vi "KT15 UP & DOWN.vi"() -> ()   [LabVIEW 2016]
uses:
  <vilib>/Instr/_visa.llb/VISA Configure Serial Port (Instr).vi
panel:
  in  "flow control 2":u16(ring) items=["None"=0, "XON/XOFF"=1, "RTS/CTS"=2, "DTR/DSR"=4]
  in  "stop bits 2":u16(ring)=10 items=["1.0"=10, "1.5"=15, "2.0"=20]
  in  "parity 2":u16(ring) items=["None", "Odd", "Even", "Mark", "Space"]
  in  "data bits 2":u16=8 min=5 max=8 step=1
  in  "KT-15 SKY":refnum<visa-resource-name>="COM17"
  in  "baud rate 2":u32=19200 min=2400 max=19200 step=2400
  out "KT-15 SKY Ambient Temperature":string
  out "KT-15 SKY  Temperature":string
  in  "Start or Stop Program":bool=TRUE
  out "KT-15 SEA Ambient Temperature":string
  out "KT-15 SEA Temperature":string
  in  "flow control":u16(ring) items=["None"=0, "XON/XOFF"=1, "RTS/CTS"=2, "DTR/DSR"=4]
  in  "stop bits":u16(ring)=10 items=["1.0"=10, "1.5"=15, "2.0"=20]
  in  "parity":u16(ring) items=["None", "Odd", "Even", "Mark", "Space"]
  in  "data bits":u16=8 min=5 max=8 step=1
  in  "KT-15 SEA":refnum<visa-resource-name>="COM16"
  in  "baud rate":u32=19200 min=2400 max=19200 step=2400
  # "COMM Port settings"
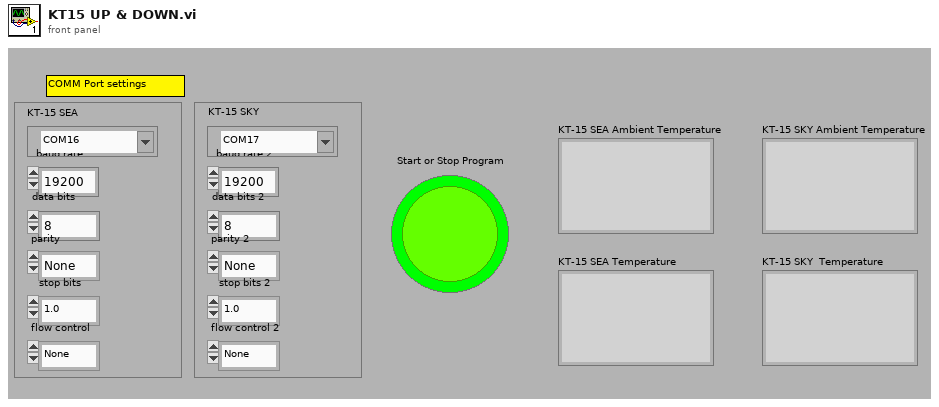
[diagram p1: front panel]
types:
  T1 = enum16{"open", "replace", "create", "open or create", "replace or create", "replace or create with confirmation"}
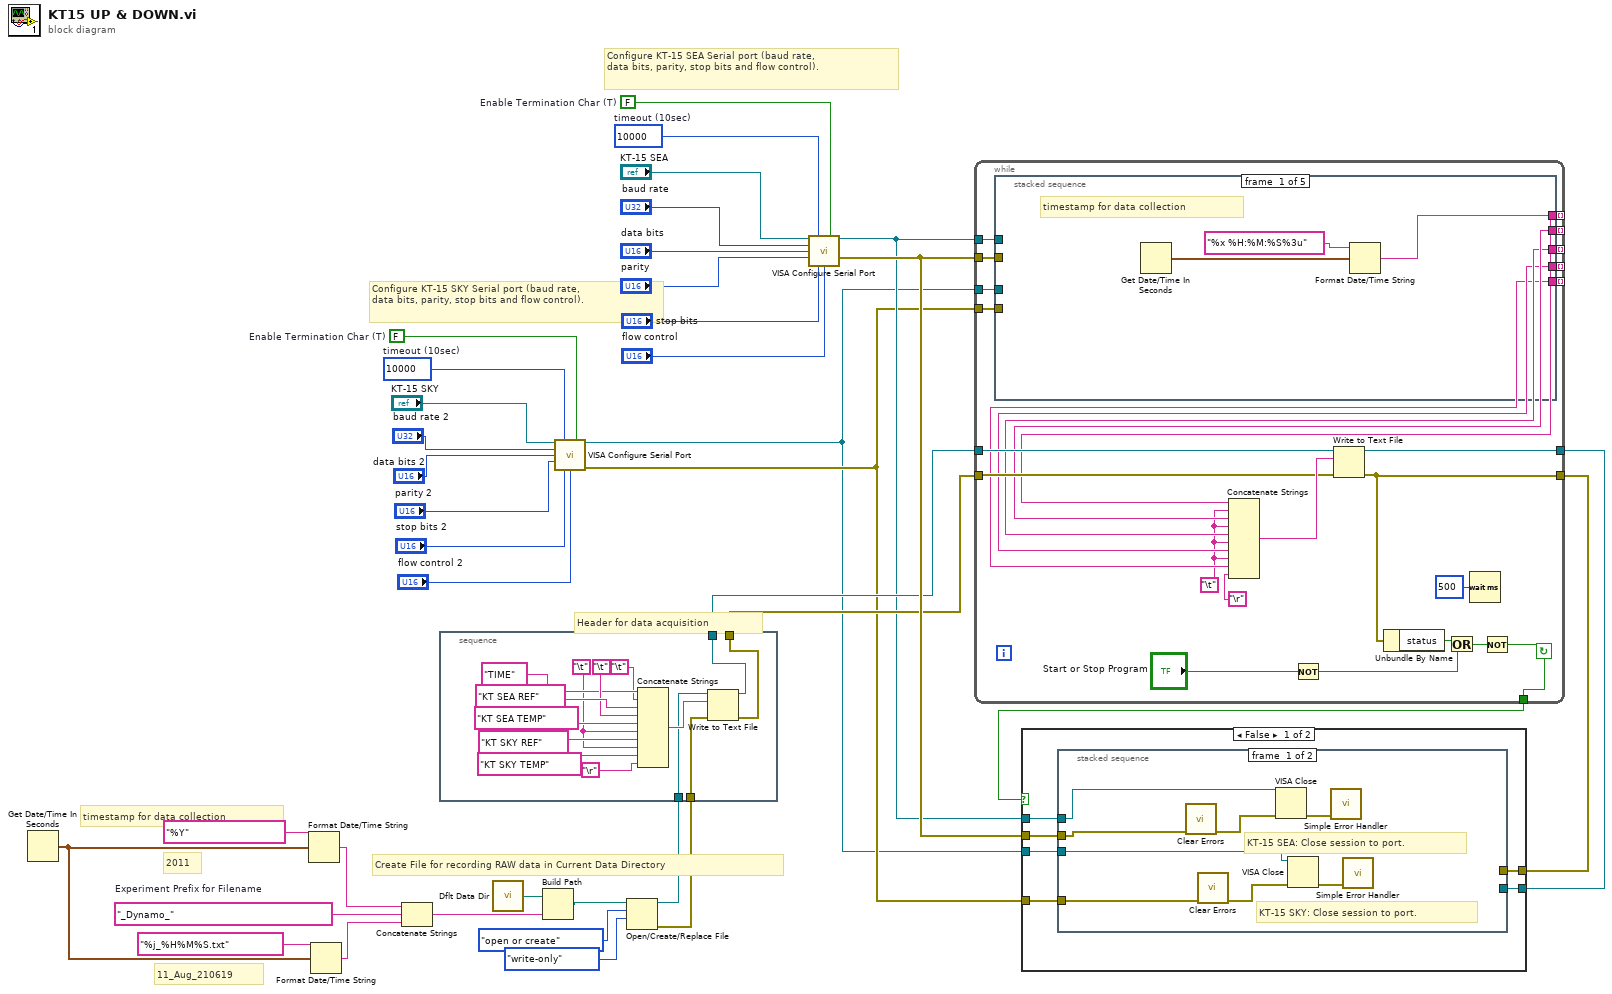
[diagram p0: block diagram]
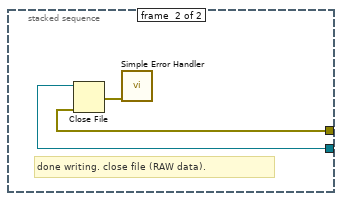
[diagram p2: hidden frame]
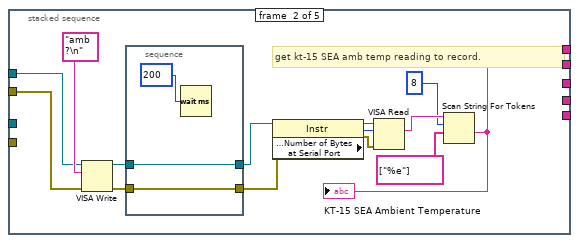
[diagram p4: hidden frame]
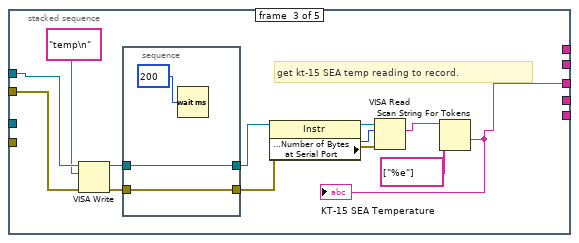
[diagram p5: hidden frame]
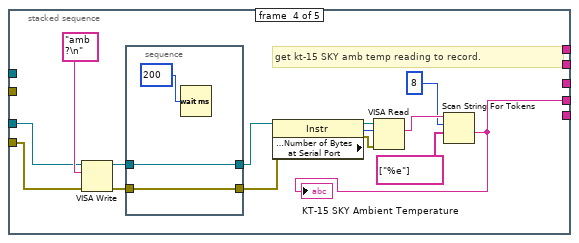
[diagram p6: hidden frame]
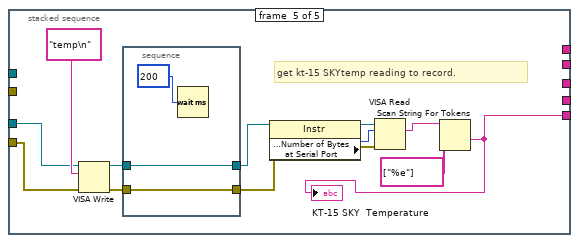
[diagram p7: hidden frame]
diagram:
  w19 = FALSE  # Enable Termination Char (T)
  w18 = u32 10000  # timeout (10sec)
  w8 = "_Dynamo_"  # Experiment Prefix for Filename
  w34 = FALSE  # Enable Termination Char (T)
  w35 = u32 10000  # timeout (10sec)
  # "2011"
  # "11_Aug_210619"
  # "timestamp for data collection"
  # "Configure KT-15 SKY Serial port (baud rate,\ndata bits, parity, stop bits and flow control)."
  # "Header for data acquisition"
  # "Create File for recording RAW data in Current Data Directory"
  # "Configure KT-15 SEA Serial port (baud rate,\ndata bits, parity, stop bits and flow control)."
  n1 = Get Date/Time In Seconds() -> (seconds since 1Jan1904=w5:timestamp)
  n2 = Format Date/Time String(time format string (%c)="%Y", seconds (now)=w5) -> (date/time string=w4:string)  [unwired: 1 out]
  n3 = Format Date/Time String(time format string (%c)="%j_%H%M%S.txt", seconds (now)=w5) -> (date/time string=w7:string)  [unwired: 1 out]
  n4 = Concatenate Strings(w4, w8, w7) -> (w1:string)
  n5 = call <vilib>:"Dflt Data Dir.vi"() -> ("App:Default Data Directory"=w3:path)
  n6 = Build Path(base path=w3, name or relative path=w1) -> (appended path=w2:path)
  n7 = call-poly "VISA Configure Serial Port"("VISA resource name"="KT-15 SKY", "timeout (10sec)"=w18, "Enable Termination\nChar (T)"=w19, "baud rate (9600)"="baud rate 2", "data bits (8)"="data bits 2", "parity (0:none)"="parity 2", "stop bits (10: 1 bit)"="stop bits 2", "flow control (0:none)"="flow control 2") -> ("VISA resource name out"=w10:refnum<visa-resource-name>, "error out"=w11:errorcluster)  [unwired: 1 in, 5 out]
  n8 = Open/Create/Replace File(file path (use dialog)=w2, operation (0:open)=T1."open or create", access (0:read/write)=enum16{"read/write", "read-only", "write-only"}."write-only") -> (refnum out=w28:refnum<file>, error out=w27:errorcluster)  [unwired: 3 in, 1 out]
  n9 = stacked-sequence {
    tunnel: w28 -> [w48]
    tunnel: w27 -> [w47]
    tunnel: [w46] -> w23
    tunnel: [w45] -> w22
    frame #0 {
      w41 = "\t"
      n10 = Concatenate Strings("TIME", "\t", "KT SEA REF", "\t", "KT SEA TEMP", w41, "KT SKY REF", w41, "KT SKY TEMP", "\r") -> (w49:string)
      n11 = Write to Text File(file (use dialog)=w48, text=w49, error in=w47) -> (refnum out=w46:refnum<file>, error out=w45:errorcluster)  [unwired: 1 in, 1 out]
    }
  }
  n12 = call-poly "VISA Configure Serial Port"("VISA resource name"="KT-15 SEA", "timeout (10sec)"=w35, "Enable Termination\nChar (T)"=w34, "baud rate (9600)"="baud rate", "data bits (8)"="data bits", "parity (0:none)"="parity", "stop bits (10: 1 bit)"="stop bits", "flow control (0:none)"="flow control") -> ("VISA resource name out"=w21:refnum<visa-resource-name>, "error out"=w24:errorcluster)  [unwired: 1 in, 5 out]
  n13 = while {
    tunnel: [w74] -> w26
    tunnel: [w73] -> w25
    tunnel: w23 -> [w68]
    tunnel: w22 -> [w67]
    tunnel: w21 -> [w71]
    tunnel: w24 -> [w70]
    tunnel: [w66] -> _ mode=indexing
    tunnel: [w65] -> _ mode=indexing
    tunnel: [w64] -> _ mode=indexing
    tunnel: [w59] -> w20
    tunnel: w10 -> [w58]
    tunnel: w11 -> [w57]
    tunnel: [w56] -> _ mode=indexing
    tunnel: [w55] -> _ mode=indexing
    stop <- w59 continue-if-true
    w53 = "\t"
    n14 = stacked-sequence {
      tunnel: [_ _ w96 _ _] -> w64
      tunnel: w71 -> [_ w86 w107 _ _]
      tunnel: w70 -> [_ w85 w106 _ _]
      tunnel: [_ w79 _ _ _] -> w65
      tunnel: [w76 _ _ _ _] -> w66
      tunnel: w58 -> [_ _ _ w113 w130]
      tunnel: w57 -> [_ _ _ w112 w129]
      tunnel: [_ _ _ w111 _] -> w56
      tunnel: [_ _ _ _ w128] -> w55
      frame #0 {
        # "timestamp for data collection"
        n15 = Get Date/Time In Seconds() -> (seconds since 1Jan1904=w77:timestamp)
        n16 = Format Date/Time String(time format string (%c)="%x %H:%M:%S%3u", seconds (now)=w77) -> (date/time string=w76:string)  [unwired: 1 out]
      }
      frame #1 {
        # "get kt-15 SEA amb temp reading to record."
        n17 = VISA Write(VISA resource name=w86, write buffer="amb ?\n", error in (no error)=w85) -> (VISA resource name out=w90:refnum<visa-resource-name>, error out=w89:errorcluster)  [unwired: 1 out]
        n18 = stacked-sequence {
          tunnel: w90 -> [w93]
          tunnel: [w93] -> w88
          tunnel: w89 -> [w92]
          tunnel: [w92] -> w87
          frame #0 {
            n19 = Wait (ms)(milliseconds to wait=u32 200 ("delay before read (ms) for AMB 2")) -> ()  [unwired: 1 out]
          }
        }
        n20 = property class="Instr"(reference=w88, error in=w87) -> (reference out=w84:refnum<visa-resource-name>, error out=w82:errorcluster, "Serial Settings:Number of Bytes at Serial Port"=w83:u32)
        n21 = VISA Read(VISA resource name=w84, byte count=w83, error in (no error)=w82) -> (read buffer=w81:string)  [unwired: 3 out]
        n22 = Scan String For Tokens(7:string[] ["%e"] ("operators (none)"), 8:8, 9:w81) -> (1:w79:string)  [unwired: 6 out]
        "KT-15 SEA Ambient Temperature" <- w79
      }
      frame #2 {
        # "get kt-15 SEA temp reading to record."
        n23 = VISA Write(VISA resource name=w107, write buffer="temp\n", error in (no error)=w106) -> (VISA resource name out=w104:refnum<visa-resource-name>, error out=w103:errorcluster)  [unwired: 1 out]
        n24 = stacked-sequence {
          tunnel: w104 -> [w109]
          tunnel: [w109] -> w101
          tunnel: w103 -> [w108]
          tunnel: [w108] -> w100
          frame #0 {
            n25 = Wait (ms)(milliseconds to wait=u32 200 ("delay before read (ms) for AMB 2")) -> ()  [unwired: 1 out]
          }
        }
        n26 = property class="Instr"(reference=w101, error in=w100) -> (reference out=w102:refnum<visa-resource-name>, error out=w99:errorcluster, "Serial Settings:Number of Bytes at Serial Port"=w98:u32)
        n27 = VISA Read(VISA resource name=w102, byte count=w98, error in (no error)=w99) -> (read buffer=w97:string)  [unwired: 3 out]
        n28 = Scan String For Tokens(7:string[] ["%e"] ("operators (none)"), 9:w97) -> (1:w96:string)  [unwired: 1 in, 6 out]
        "KT-15 SEA Temperature" <- w96
      }
      frame #3 {
        # "get kt-15 SKY amb temp reading to record."
        n29 = VISA Write(VISA resource name=w113, write buffer="amb ?\n", error in (no error)=w112) -> (VISA resource name out=w123:refnum<visa-resource-name>, error out=w122:errorcluster)  [unwired: 1 out]
        n30 = stacked-sequence {
          tunnel: w123 -> [w126]
          tunnel: [w126] -> w121
          tunnel: w122 -> [w125]
          tunnel: [w125] -> w120
          frame #0 {
            n31 = Wait (ms)(milliseconds to wait=u32 200 ("delay before read (ms) for AMB 2")) -> ()  [unwired: 1 out]
          }
        }
        n32 = property class="Instr"(reference=w121, error in=w120) -> (reference out=w119:refnum<visa-resource-name>, error out=w117:errorcluster, "Serial Settings:Number of Bytes at Serial Port"=w118:u32)
        n33 = VISA Read(VISA resource name=w119, byte count=w118, error in (no error)=w117) -> (read buffer=w116:string)  [unwired: 3 out]
        n34 = Scan String For Tokens(7:string[] ["%e"] ("operators (none)"), 8:8, 9:w116) -> (1:w111:string)  [unwired: 6 out]
        "KT-15 SKY Ambient Temperature" <- w111
      }
      frame #4 {
        # "get kt-15 SKYtemp reading to record."
        n35 = VISA Write(VISA resource name=w130, write buffer="temp\n", error in (no error)=w129) -> (VISA resource name out=w139:refnum<visa-resource-name>, error out=w138:errorcluster)  [unwired: 1 out]
        n36 = stacked-sequence {
          tunnel: w139 -> [w142]
          tunnel: [w142] -> w136
          tunnel: w138 -> [w141]
          tunnel: [w141] -> w135
          frame #0 {
            n37 = Wait (ms)(milliseconds to wait=u32 200 ("delay before read (ms) for AMB 2")) -> ()  [unwired: 1 out]
          }
        }
        n38 = property class="Instr"(reference=w136, error in=w135) -> (reference out=w137:refnum<visa-resource-name>, error out=w134:errorcluster, "Serial Settings:Number of Bytes at Serial Port"=w133:u32)
        n39 = VISA Read(VISA resource name=w137, byte count=w133, error in (no error)=w134) -> (read buffer=w132:string)  [unwired: 3 out]
        n40 = Scan String For Tokens(7:string[] ["%e"] ("operators (none)"), 9:w132) -> (1:w128:string)  [unwired: 1 in, 6 out]
        "KT-15 SKY  Temperature" <- w128
      }
    }
    n41 = Concatenate Strings(w66, w53, w65, w53, w64, w53, w56, w53, w55, "\r") -> (w69:string)
    n42 = Not(x="Start or Stop Program") -> (.not. x?=w60:bool)
    n43 = Write to Text File(file (use dialog)=w68, text=w69, error in=w67) -> (refnum out=w74:refnum<file>, error out=w73:errorcluster)  [unwired: 1 in, 1 out]
    n44 = Unbundle By Name(w73) -> ("status"=w63:bool)
    n45 = Or(x=w63, y=w60) -> (x .or. y?=w61:bool)
    n46 = Wait (ms)(milliseconds to wait=u32 500 ("millisecond multiple")) -> ()  [unwired: 1 out]
    n47 = Not(x=w61) -> (.not. x?=w59:bool)
  }
  n48 = case shown="False" w20 {
    tunnel: w21 -> [w149 _]
    tunnel: w24 -> [w148 _]
    tunnel: w26 -> [w146 _]
    tunnel: w25 -> [w147 _]
    tunnel: w11 -> [w145 _]
    tunnel: w10 -> [w144 _]
    frame False {
      n49 = stacked-sequence {
        tunnel: w149 -> [w155 _]
        tunnel: w148 -> [w154 _]
        tunnel: w147 -> [_ w159]
        tunnel: w146 -> [_ w158]
        tunnel: w145 -> [w151 _]
        tunnel: w144 -> [w150 _]
        frame #0 {
          # "KT-15 SKY: Close session to port."
          # "KT-15 SEA: Close session to port."
          n50 = call <vilib>:"Clear Errors.vi"("error in (no error)"=w154) -> ("error out"=w156:errorcluster)  [unwired: 1 in, 5 out]
          n51 = call <vilib>:"Clear Errors.vi"("error in (no error)"=w151) -> ("error out"=w152:errorcluster)  [unwired: 1 in, 5 out]
          n52 = VISA Close(VISA resource name=w155, error in (no error)=w156) -> (error out=w157:errorcluster)
          n53 = VISA Close(VISA resource name=w150, error in (no error)=w152) -> (error out=w153:errorcluster)
          n54 = call <vilib>:"Simple Error Handler.vi"("error in (no error)"=w157) -> ()  [unwired: 1 in, 8 out]
          n55 = call <vilib>:"Simple Error Handler.vi"("error in (no error)"=w153) -> ()  [unwired: 1 in, 8 out]
        }
        frame #1 {
          # "done writing. close file (RAW data)."
          n56 = Close File(refnum=w158, error in=w159) -> (error out=w160:errorcluster)  [unwired: 1 out]
          n57 = call <vilib>:"Simple Error Handler.vi"("error in (no error)"=w160) -> ()  [unwired: 1 in, 8 out]
        }
      }
    }
    frame True {
    }
  }
